vi "BRig_dataExp_Audio_freq_L.vi"() -> (2 "output_Audio_freq__L":i32)   [LabVIEW 2014]
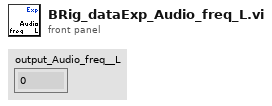
[diagram p1: front panel]
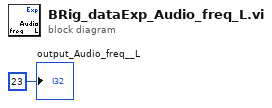
[diagram p0: block diagram]
diagram:
  "output_Audio_freq__L" <- 23 ("output_iBlock")
